vi "Get Context.vi"(8 "error in (no error)":errorcluster, 11 "Process In":refnum<class "Process.lvclass">) -> (0 "error out":errorcluster, 2 "Context":refnum<class "Process.lvclass">, 3 "Process Out":refnum<class "Process.lvclass">)   [LabVIEW 2020, in "Process.lvclass"]
doc: "Returns the context of the process. If the process is top level application an error is returned."
uses:
  Process.lvclass
  Process.lvclass/Process.ctl
  <vilib>/Utility/error.llb/Clear Errors.vi
  <vilib>/Utility/error.llb/Error Cluster From Error Code.vi
  <vilib>/ErrorRing/Error Ring.xnode
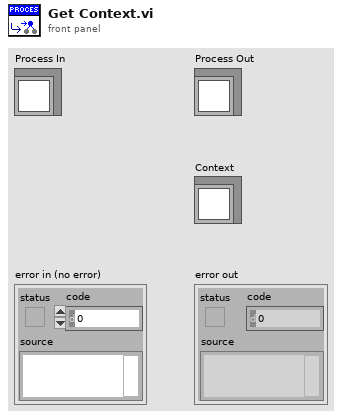
[diagram p1: front panel]
types:
  T1 = typedef "Process.lvclass/Lifecycle State.ctl" = enum16{"Uninitialized", "Initialized", "Started", "Running", "Stopped", "Finished"}
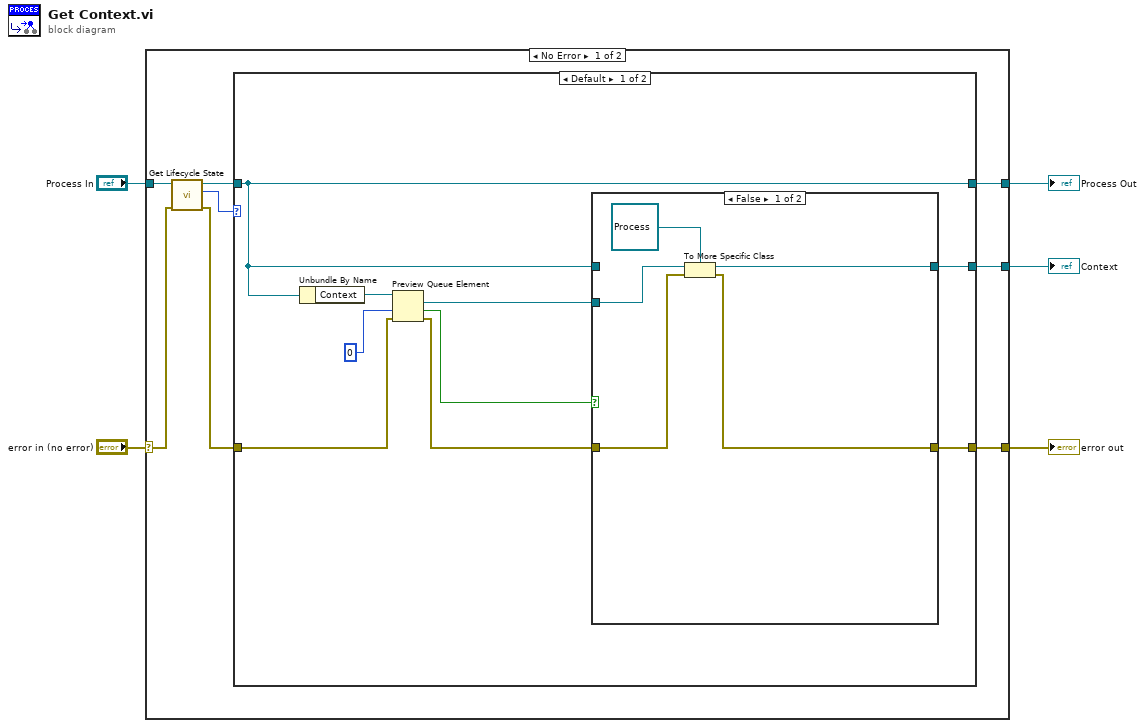
[diagram p0: block diagram]
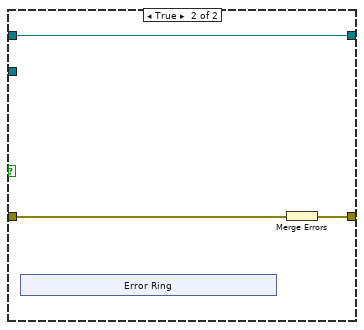
[diagram p2: hidden frame]
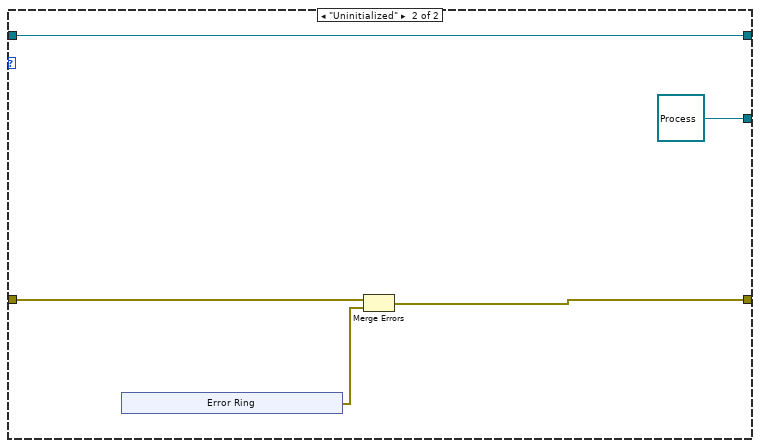
[diagram p3: hidden frame]
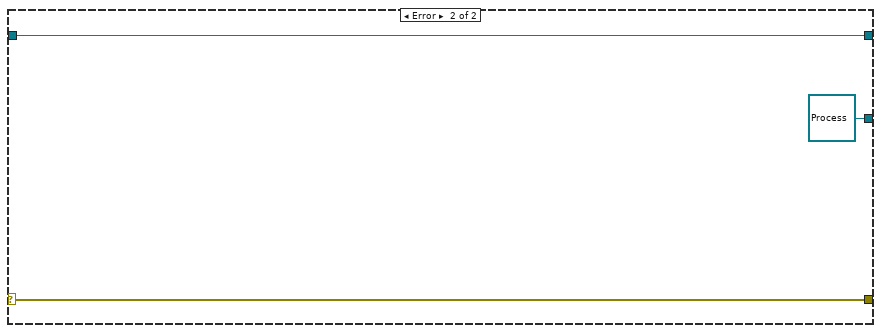
[diagram p4: hidden frame]
diagram:
  n1 = case shown="No Error" "error in (no error)" {
    selector: "error in (no error)" -> [w8 w46]
    tunnel: "Process In" -> [w13 w45]
    tunnel: [w12 w45] -> w4
    tunnel: [w11 refnum<class "Process.lvclass"> refnum ("Error Handler")] -> w3
    tunnel: [w10 w46] -> w2
    frame No Error {
      n2 = call "Get Lifecycle State.vi"("error in (no error)"=w8, "Process In"=w13) -> ("error out"=w7:errorcluster, "Lifecycle State"=w6:T1, "Process Out"=w9:refnum<class "Process.lvclass">)  [unwired: 6 in, 1 out]
      n3 = case shown="Default" w6 {
        tunnel: w9 -> [w14 w37]
        tunnel: [w14 w37] -> w12
        tunnel: [w22 refnum<class "Process.lvclass"> refnum ("Error Handler")] -> w11
        tunnel: [w21 w36] -> w10
        tunnel: w7 -> [w16 w39]
        frame Default {
          n4 = Unbundle By Name(w14) -> ("Context"=w20:refnum<queue>)
          n5 = Preview Queue Element(queue=w20, timeout in ms (-1)=0, error in (no error)=w16) -> (element=w17:refnum<class>, timed out?=w15:bool, error out=w19:errorcluster)  [unwired: 1 out]
          n6 = case shown="False" w15 {
            tunnel: [w27 w28] -> w22
            tunnel: [w23 w29] -> w21
            tunnel: w17 -> [w25 _]
            tunnel: w19 -> [w24 w30]
            tunnel: w14 -> [_ w28]
            frame False {
              n7 = To More Specific Class(target class=refnum<class "Process.lvclass"> refnum ("Error Handler"), reference=w25, error in=w24) -> (specific class reference=w27:refnum<class "Process.lvclass">, error out=w23:errorcluster)
            }
            frame True {
              n8 = xnode "Error Ring"() -> ()  [unwired: 1 out]
              n9 = Merge Errors(w30) -> (w29:errorcluster)
            }
          }
        }
        frame "Uninitialized" {
          n10 = xnode "Error Ring"() -> ("error out"=w35:errorcluster)
          n11 = Merge Errors(w39, w35) -> (w36:errorcluster)
        }
      }
    }
    frame Error {
    }
  }
  "error out" <- w2
  "Process Out" <- w4
  "Context" <- w3
